vi "Initialize Modules.vi"(8 "error in (no error)":errorcluster, 10 "Modules":refnum<class "Module.lvclass">[](array[class]), 11 "Block Diagram in":refnum<class "Block Diagram.lvclass">) -> (0 "error out":errorcluster, 3 "Block Diagram out":refnum<class "Block Diagram.lvclass">)   [LabVIEW 2015, in "Block Diagram.lvclass"]
uses:
  Block Diagram.lvclass
  Module/Module Class/Module.lvclass
  Block Diagram.lvclass/Block Diagram.ctl
  Initial Sequence/Initial Sequence.lvclass
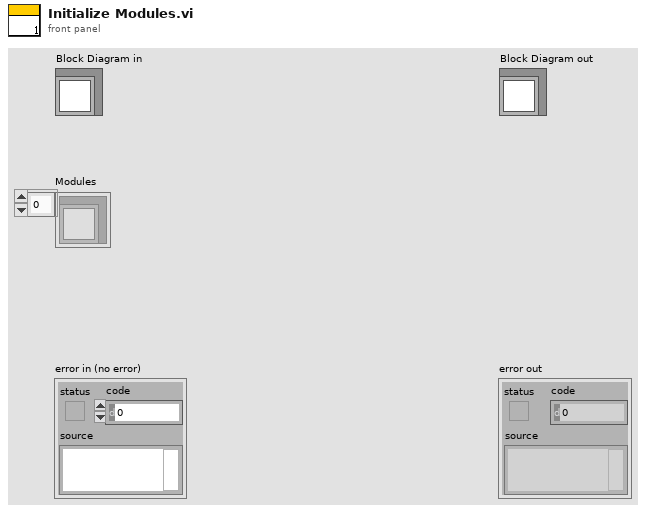
[diagram p1: front panel]
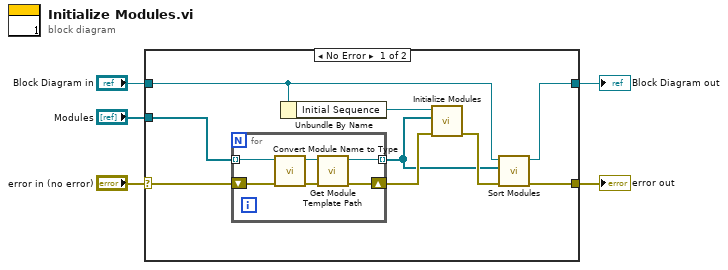
[diagram p0: block diagram]
diagram:
  n1 = case shown="No Error" "error in (no error)" {
    selector: "error in (no error)" -> [w12 w22]
    tunnel: [w9 w22] -> w4
    tunnel: [w6 w21] -> w2
    tunnel: "Block Diagram in" -> [w7 w21]
    tunnel: "Modules" -> [w13 _]
    frame No Error {
      n2 = for {
        tunnel: w13 -> [w20] mode=indexing
        tunnel: [w18] -> w8 mode=indexing
        shift-right: [w17] -> w11
        shift-left: w12 -> [w15]
        n3 = call "Convert Module Name to Type.vi"("error in (no error)"=w15, "Module in"=w20) -> ("error out"=w16:errorcluster, "Module out"=w19:refnum<class "Module.lvclass">)  [unwired: 8 in]
        n4 = call-dynamic "Get Module Template Path.vi"("error in (no error)"=w16, "Module in"=w19) -> ("error out"=w17:errorcluster, "Module out"=w18:refnum<class "Module.lvclass">)  [unwired: 8 in]
      }
      n5 = Unbundle By Name(w7) -> ("Initial Sequence"=w14:refnum<class "Initial Sequence.lvclass">)
      n6 = call "Initialize Modules.vi"("error in (no error)"=w11, "Modules"=w8, "Initial Sequence in"=w14) -> ("error out"=w10:errorcluster)  [unwired: 7 in, 1 out]
      n7 = call "Sort Modules.vi"("error in (no error)"=w10, "Modules"=w8, "Block Diagram in"=w7) -> ("error out"=w9:errorcluster, "Block Diagram out"=w6:refnum<class "Block Diagram.lvclass">)  [unwired: 7 in]
    }
    frame Error {
    }
  }
  "error out" <- w4
  "Block Diagram out" <- w2
